vi "Units_RotationsPerMinuteToRadiansPerSecond.vi"(10 "RotationsPerMinute":dbl) -> (2 "RadiansPerSecond":dbl)   [LabVIEW 2019, in "Trajectory_Library.lvlib"]
doc: "Convert a value from revolutions per minute (RPM) to radians/sec \n\nInputs: \n - RevolutionsPerMinute - Speed ( RPM )\n\nOutputs:\n - RadiansPerSec - Speed (Radians / Second)"
uses:
  Trajectory_Library.lvlib
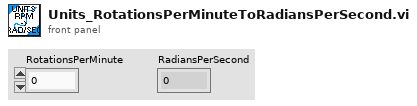
[diagram p1: front panel]
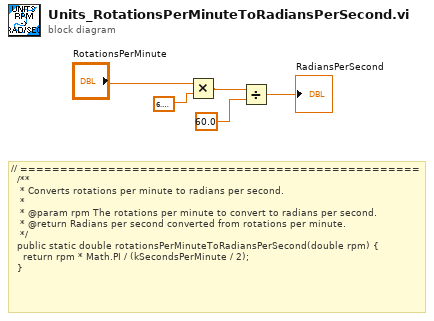
[diagram p0: block diagram]
diagram:
  # "// ==================================================\n  /**\n   * Converts rotations per minute to radians per second.\n   *\n   * @param rpm The rotations per minute to convert to radians per second.\n   * @return Radians per second converted from rotations per minute.\n   */\n  public static double rotationsPerMinuteToRadiansPerSecond(double rpm) {\n    return rpm * Math.PI / (kSecondsPerMinute / 2);\n  }"
  n1 = Multiply(x="RotationsPerMinute", y=6.283185307179586) -> (x*y=w2:dbl)
  n2 = Divide(x=w2, y=60.0) -> (x/y=→"RadiansPerSecond":dbl)
